vi "ni5660 Initiate IQ.vi"(0 "receiver info in":T1, 11 "error in (no error)":errorcluster) -> (4 "receiver info out":T1, 15 "error out":errorcluster)   [LabVIEW 2011]
doc: "This VI initiates an IQ waveform acquisition. Use this VI with ni5660 Fetch IQ VI when performing finite or continuous acquisition."
uses:
  <vilib>/addons/Modulation/niScope/controls/mod_Modulation Settings.ctl
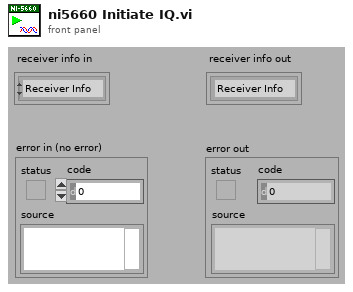
[diagram p1: front panel]
types:
  T1 = typedef "mod_Modulation Settings.ctl" = cluster{enum16{"Receiver Info"}, variant}
  T2 = typedef "mod_Readable Attributes Cluster.ctl" = cluster{"carrier":cluster{"frequency":dbl}, "receiver":cluster{"handles":cluster{"niTuner taskID":i32, "niScope handle":refnum<k15>}, "RFSA":cluster{"reference level":i32, "RF attenuation":i32}, "data format":enum16{"real", "complex modulated (array)", "complex modulated (interleaved)"}, "auto suppress SW IQ":enum16{"off", "on"}, "IQ sample rate":dbl, "bandwidth":dbl}}
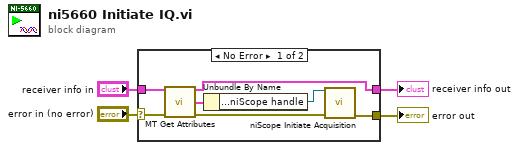
[diagram p0: block diagram]
diagram:
  n1 = case shown="No Error" "error in (no error)" {
    selector: "error in (no error)" -> [w8 w12]
    tunnel: "receiver info in" -> [w9 w13]
    tunnel: [w5 w12] -> w3
    tunnel: [w7 w13] -> w1
    frame No Error {
      n2 = call <vilib>:"MT Get Attributes.vi"("receiver info in"=w9, "error in (no error)"=w8) -> ("receiver info out"=w7:T1, "attributes"=w11:T2, "error out"=w10:errorcluster)  [unwired: 11 in]
      n3 = Unbundle By Name(w11) -> ("receiver.handles.niScope handle"=w6:refnum<k15>)
      n4 = call <instrlib>:"niScope Initiate Acquisition.vi"("instrument handle"=w6, "error in"=w10) -> ("error out"=w5:errorcluster)  [unwired: 12 in, 1 out]
    }
    frame Error {
    }
  }
  "error out" <- w3
  "receiver info out" <- w1
